vi "BitsPerPixel.vi"(1 "camera cluster":T3) -> (0 "BitsPerPixel":u32)   [LabVIEW 2015]
uses:
  <vilib>/vision/Avi1.llb/AviRefnum.ctl
  <vilib>/userdefined/High Color/IMAQdx.ctl
  <vilib>/vision/driver/NI_Vision_Acquisition_Software.lvlib
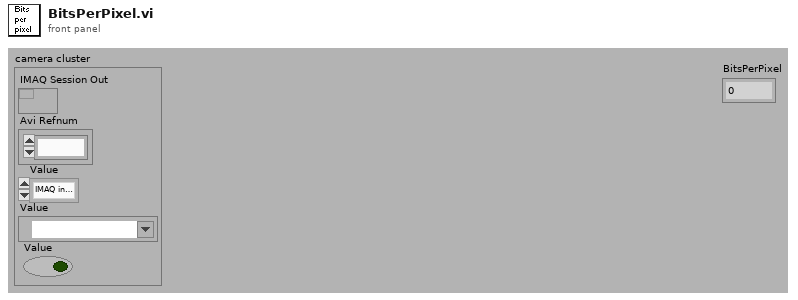
[diagram p1: front panel]
types:
  T1 = typedef "AviRefnum.ctl" = refnum<k1>
  T2 = typedef "IMAQdx.ctl" = refnum<k21>
  T3 = cluster{"IMAQ Session Out":refnum<k11>, "Avi Refnum":T1, "Value":enum32{"IMAQ interface", "IMAQdx interface", "AVI file"}, "Value":T2, "Value":bool}
  T4 = enum32{"IMAQ interface", "IMAQdx interface", "AVI file"}
  T5 = typedef "IMAQ Image.ctl" = refnum<image>
  T6 = typedef "Image Type" = u32
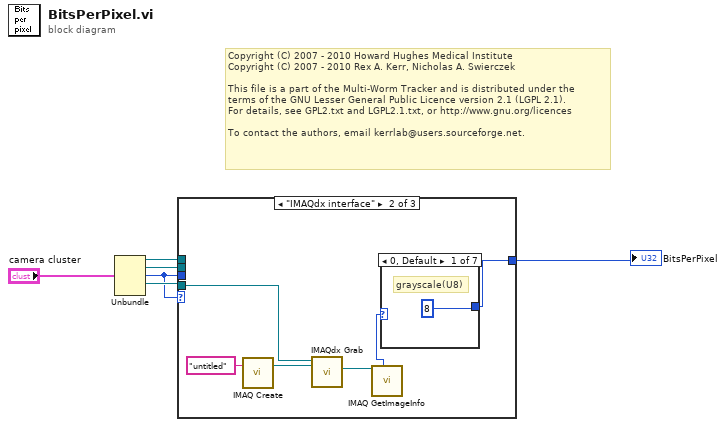
[diagram p0: block diagram]
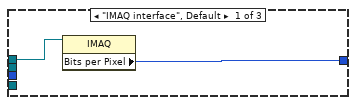
[diagram p2: hidden frame]
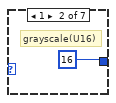
[diagram p3: hidden frame]
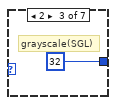
[diagram p4: hidden frame]
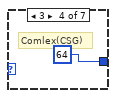
[diagram p5: hidden frame]
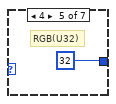
[diagram p6: hidden frame]
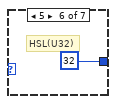
[diagram p7: hidden frame]
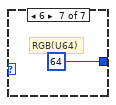
[diagram p8: hidden frame]
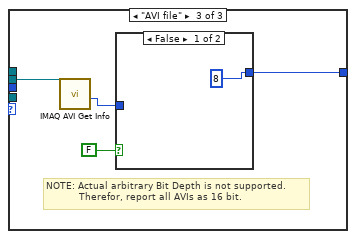
[diagram p9: hidden frame]
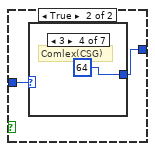
[diagram p10: hidden frame]
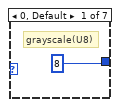
[diagram p11: hidden frame]
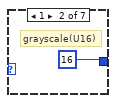
[diagram p12: hidden frame]
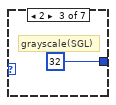
[diagram p13: hidden frame]
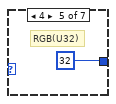
[diagram p14: hidden frame]
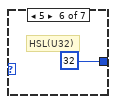
[diagram p15: hidden frame]
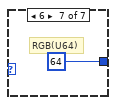
[diagram p16: hidden frame]
diagram:
  # "Copyright (C) 2007 - 2010 Howard Hughes Medical Institute\nCopyright (C) 2007 - 2010 Rex A. Kerr, Nicholas A. Swierczek\n \nThis file is a part of the Multi-Worm Tracker and is distributed under the\nterms of the GNU Lesser General Public Licence version 2.1 (LGPL 2.1).\nFor details, see GPL2.txt and LGPL2.1.txt, or http://www.gnu.org/licences\n \nTo contact the authors, email kerrlab@users.sourceforge.net."
  n1 = Unbundle("camera cluster") -> ("IMAQ Session Out"=w6:refnum<k11>, "Avi Refnum"=w3:T1, "Value"=w2:T4, "Value"=w4:T2)  [unwired: 1 out]
  n2 = case shown="\"IMAQdx interface\"" w2 {
    tunnel: w4 -> [_ w11 _]
    tunnel: w6 -> [w8 _ _]
    tunnel: [w7 w14 w24] -> w5
    tunnel: w2 -> [_ _ _]
    tunnel: w3 -> [_ _ w22]
    frame "IMAQ interface", Default {
      n3 = property class="IMAQ"(reference=w8) -> ("Bits per Pixel"=w7:u32)  [unwired: 1 in, 2 out]
    }
    frame "IMAQdx interface" {
      n4 = call "IMAQ Create"("Image Name"="untitled") -> ("New Image"=w12:T5)  [unwired: 4 in, 1 out]
      n5 = call <vilib>:"IMAQdx Grab.vi"("Image In"=w12, "Session In"=w11) -> ("Image Out"=w10:T5)  [unwired: 6 in, 3 out]
      n6 = call "IMAQ GetImageInfo"("Image"=w10) -> ("Image Type"=w9:T6)  [unwired: 3 in, 7 out]
      n7 = case shown="0, Default" w9 {
        tunnel: [8 16 32 64 32 32 64] -> w14
        frame 0, Default {
          # "grayscale(U8)"
        }
        frame 1 {
          # "grayscale(U16)"
        }
        frame 2 {
          # "grayscale(SGL)"
        }
        frame 3 {
          # "Comlex(CSG)"
        }
        frame 4 {
          # "RGB(U32)"
        }
        frame 5 {
          # "HSL(U32)"
        }
        frame 6 {
          # "RGB(U64)"
        }
      }
    }
    frame "AVI file" {
      # "NOTE: Actual arbitrary Bit Depth is not supported.\n           Therefor, report all AVIs as 16 bit."
      n8 = call "IMAQ AVI Get Info"("Avi Refnum"=w22) -> ("Image Type"=w25:T6)  [unwired: 6 in, 4 out]
      n9 = case shown="False" FALSE {
        tunnel: w25 -> [_ w28]
        tunnel: [8 w27] -> w24
        frame False {
        }
        frame True {
          n10 = case shown="3" w28 {
            tunnel: [8 16 32 64 32 32 64] -> w27
            frame 0, Default {
              # "grayscale(U8)"
            }
            frame 1 {
              # "grayscale(U16)"
            }
            frame 2 {
              # "grayscale(SGL)"
            }
            frame 3 {
              # "Comlex(CSG)"
            }
            frame 4 {
              # "RGB(U32)"
            }
            frame 5 {
              # "HSL(U32)"
            }
            frame 6 {
              # "RGB(U64)"
            }
          }
        }
      }
    }
  }
  "BitsPerPixel" <- w5
